vi "ToDatagram.vi"(8 "error in (no error)":errorcluster, 10 "messageID":u16, 11 "PublishReleaseMqttMsg in":refnum<class "PublishReleaseMqttMsg.lvclass">) -> (0 "error out":errorcluster, 2 "Datagram":u8[](array[numeric]), 3 "PublishReleaseMqttMsg out":refnum<class "PublishReleaseMqttMsg.lvclass">)   [LabVIEW 2020, in "PublishReleaseMqttMsg.lvclass"]
uses:
  PublishReleaseMqttMsg.lvclass
  BaseMqttMsg.lvclass
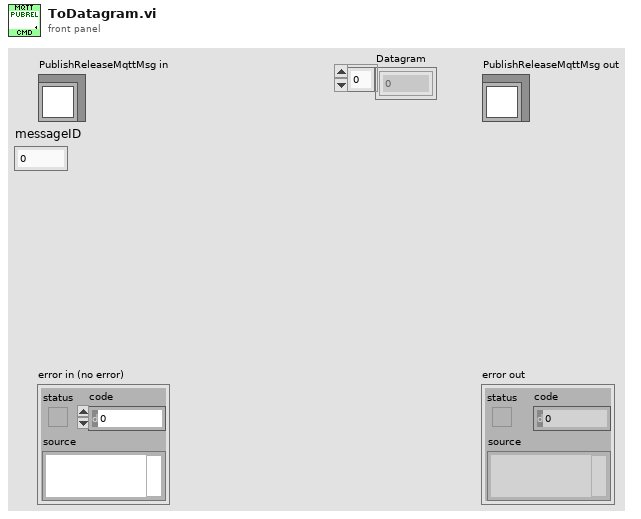
[diagram p1: front panel]
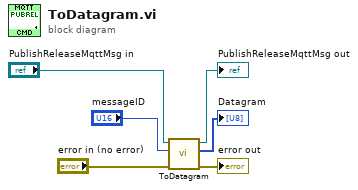
[diagram p0: block diagram]
diagram:
  n1 = call-parent "ToDatagram.vi"("error in (no error)"="error in (no error)", "messageID"="messageID", "BaseMqttMsg in"="PublishReleaseMqttMsg in") -> ("error out"=→"error out":errorcluster, "Datagram"=→"Datagram":u8[], "BaseMqttMsg out"=→"PublishReleaseMqttMsg out":refnum<class "PublishReleaseMqttMsg.lvclass">)  [unwired: 6 in]
